vi "grados_a_pasos.vi"(10 "Microstep":u32, 11 "Grados/minuto \n(goniometro)":u32) -> (2 "Velocidad motor \n(pasos/segundo)":u32)   [LabVIEW 2016]
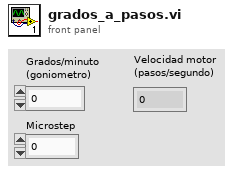
[diagram p1: front panel]
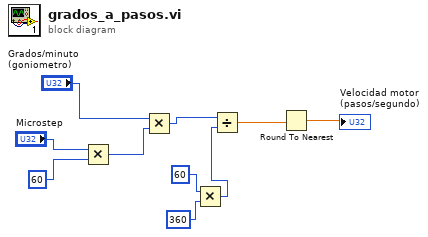
[diagram p0: block diagram]
diagram:
  n1 = Multiply(x="Microstep", y=60) -> (x*y=w9:u32)
  n2 = Multiply(x="Grados/minuto \n(goniometro)", y=w9) -> (x*y=w6:u32)
  n3 = Multiply(x=u32 60 ("y"), y=360) -> (x*y=w2:u32)
  n4 = Divide(x=w6, y=w2) -> (x/y=w5:dbl)
  n5 = Round To Nearest(number=w5) -> (nearest integer value=→"Velocidad motor \n(pasos/segundo)":dbl)
